vi "2_1.vi"() -> ()   [LabVIEW 2020]
panel:
  out "Negativ":bool
  out "Positiv":bool
  in  "Drehknopf":dbl(knob) scale=0.0..10.0
  in  "Stopp":bool
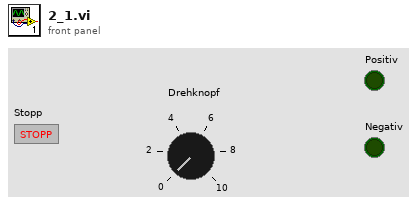
[diagram p1: front panel]
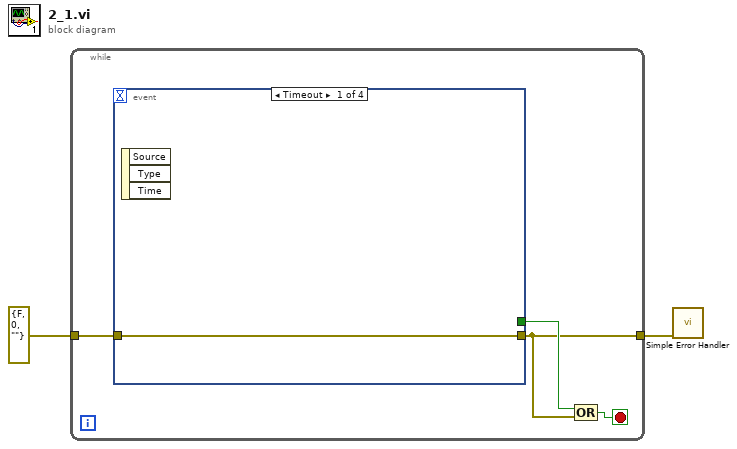
[diagram p0: block diagram]
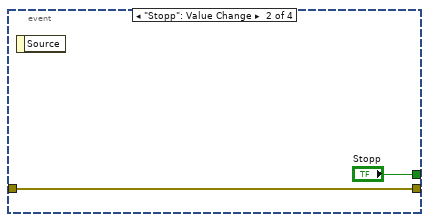
[diagram p2: hidden frame]
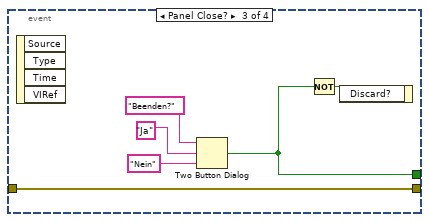
[diagram p3: hidden frame]
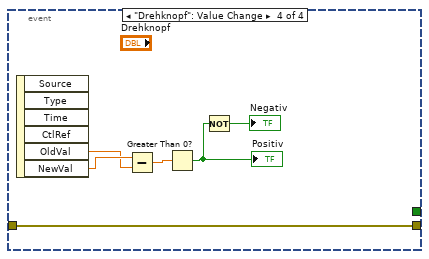
[diagram p4: hidden frame]
diagram:
  n1 = while {
    tunnel: errorcluster {"status"=FALSE, "code"=0, "source"=""} ("Fehlerkonstante") -> [w4]
    tunnel: [w3] -> w1
    stop <- w6 stop-if-true
    n2 = event shown="[0] Timeout" {
      selector: _ -> [_ _ _ _]
      dyn-events: _ -> [_ _ _ _]
      timeout: _ -> [_ _ _ _]
      tunnel: [_ "Stopp" w14 _] -> w5
      tunnel: w4 -> [w7 w8 w10 w16]
      tunnel: [w7 w8 w10 w16] -> w3
      event Timeout {
        n3 = event-data() -> ()  [unwired: 1 in, 3 out]
      }
      event "Stopp": Value Change {
        n4 = event-data() -> ()  [unwired: 1 in, 1 out]
      }
      event Panel Close? {
        n5 = event-data() -> ()  [unwired: 1 in, 4 out]
        n6 = Two Button Dialog(message="Beenden?" ("Nachricht"), 1:"Nein" ("Text für F-Schaltfläche (\"Abbrechen\")"), 2:"Ja" ("Text für T-Schaltfläche (\"OK\")")) -> (T button?=w14:bool)
        n7 = Not(x=w14) -> (.not. x?=w15:bool)
        n8 = event-data("Discard?"=w15) -> ()  [unwired: 1 in, 1 out]
      }
      event "Drehknopf": Value Change {
        n9 = event-data() -> ("OldVal"=w20:dbl, "NewVal"=w21:dbl)  [unwired: 1 in, 4 out]
        n10 = Subtract(x=w21, y=w20) -> (x-y=w19:dbl)
        n11 = Greater Than 0?(x=w19) -> (x > 0?=w18:bool)
        "Positiv" <- w18
        n12 = Not(x=w18) -> (.not. x?=→"Negativ":bool)
      }
    }
    n13 = Compound Arithmetic op=OR ("Mehrfacharithmetik")(w5, w3) -> (w6:bool)
  }
  n14 = call <vilib>:"Simple Error Handler.vi"("error in (no error)"=w1) -> ()  [unwired: 4 in, 5 out]
